vi "cm_Time Domain Display.vi"() -> ()   [LabVIEW 2009, in "Channel Monitor [System].xctl"]
uses:
  Channel Monitor [System].xctl
  <vilib>/Utility/error.llb/DialogType.ctl
panel:
  out "Waveform Graph":waveform(dbl)(graph)
  out "error out":errorcluster
  out "channel":i32
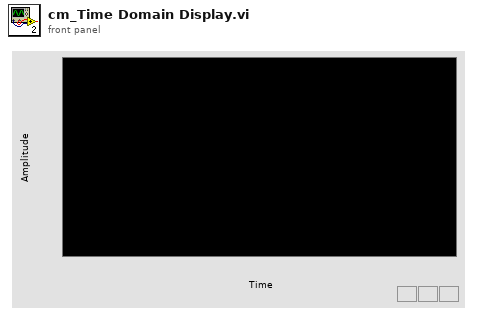
[diagram p1: front panel]
types:
  T1 = typedef "amc_Message Queue.ctl" = refnum<queue>
  T2 = typedef "DialogType.ctl" = u16
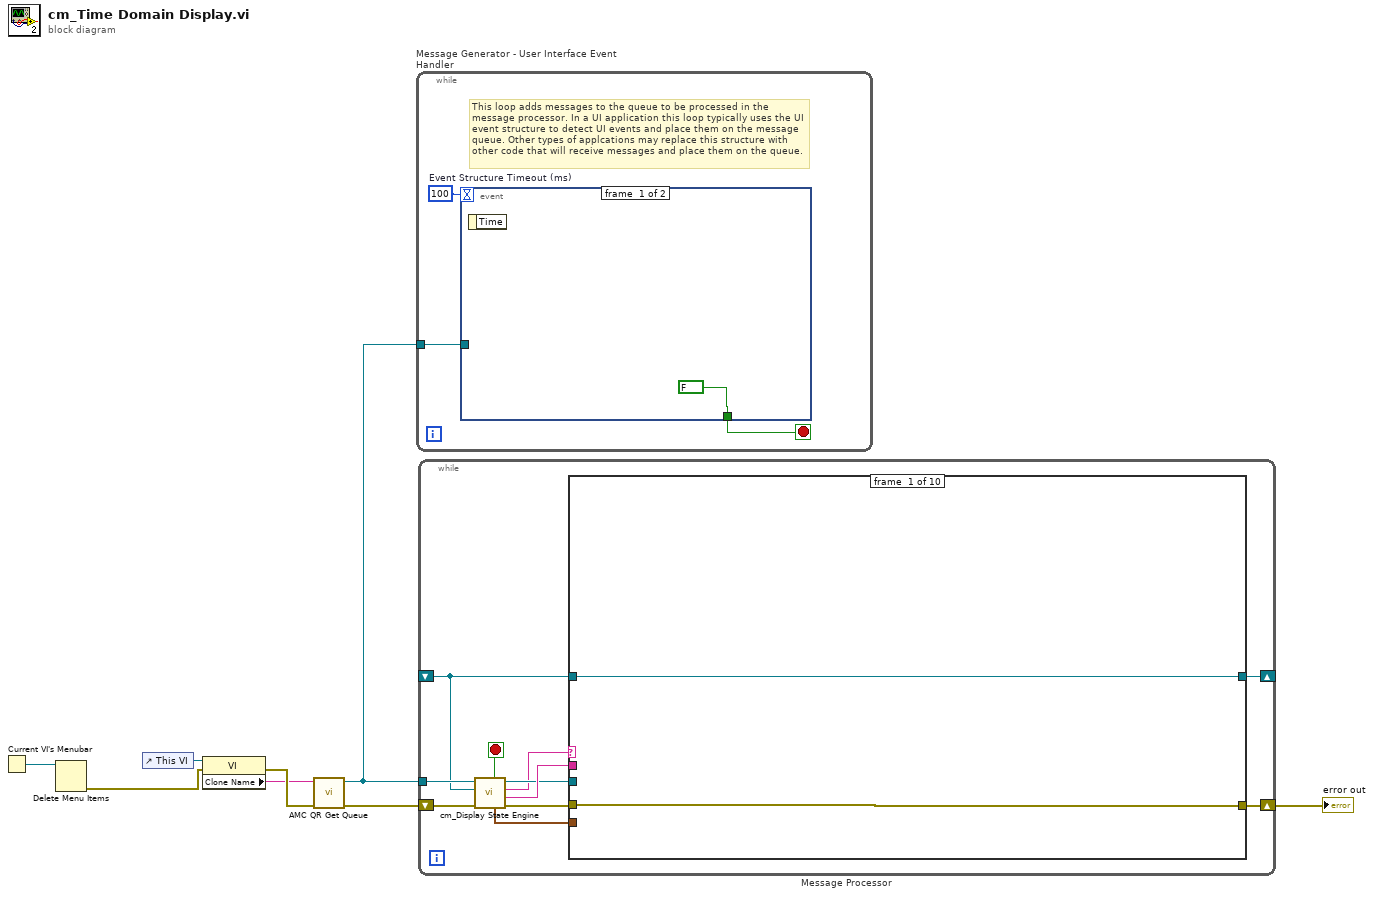
[diagram p0: block diagram]
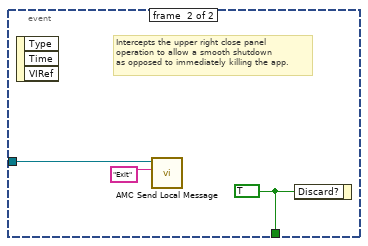
[diagram p2: hidden frame]
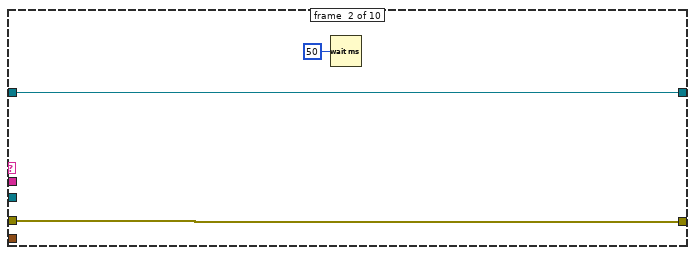
[diagram p3: hidden frame]
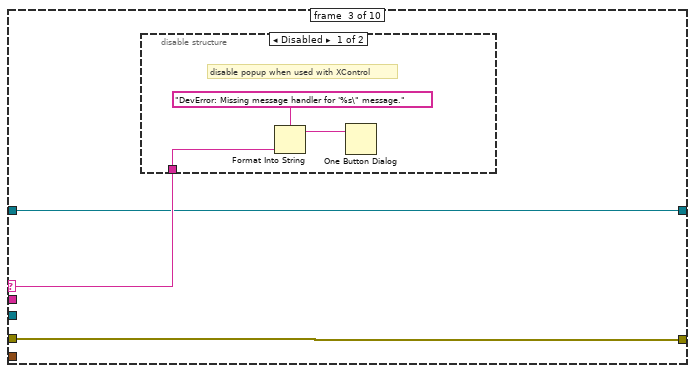
[diagram p4: hidden frame]
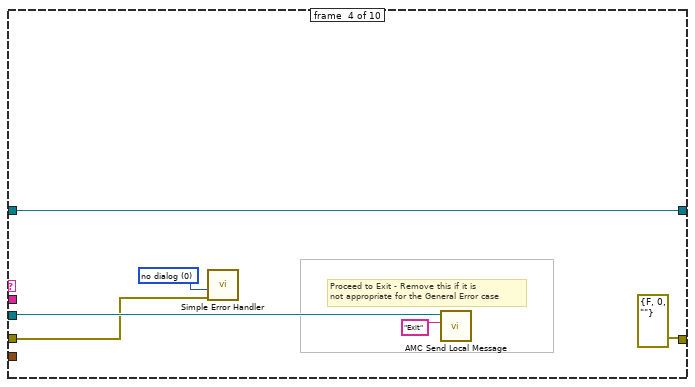
[diagram p6: hidden frame]
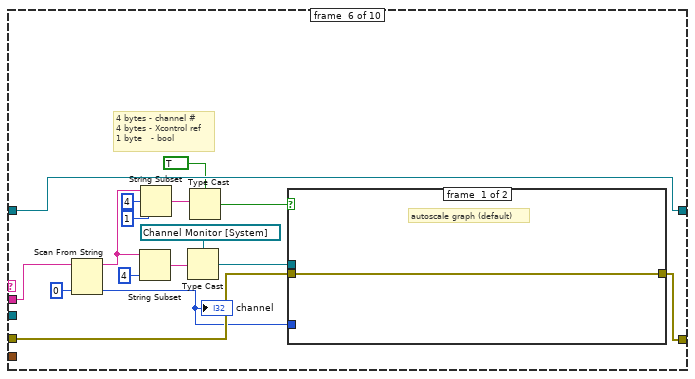
[diagram p8: hidden frame]
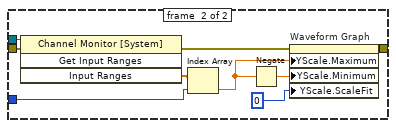
[diagram p9: hidden frame]
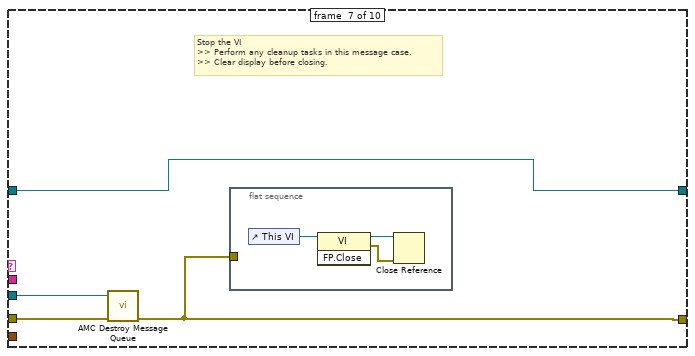
[diagram p10: hidden frame]
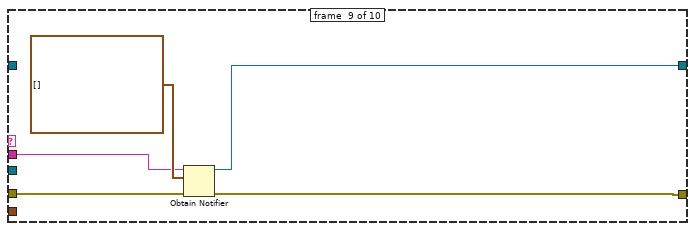
[diagram p12: hidden frame]
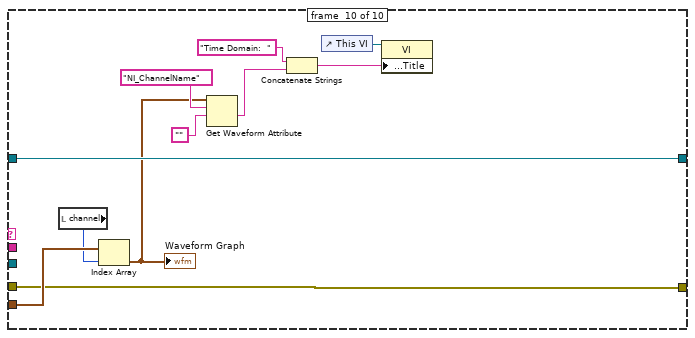
[diagram p13: hidden frame]
diagram:
  n1 = Current VI's Menubar() -> (w6:refnum<k9>)
  n2 = Delete Menu Items(9:w6) -> (0:w4:errorcluster)  [unwired: 3 in, 1 out]
  n3 = control-ref of="This VI"() -> (w7:refnum<vi>)
  n4 = property class="VI"(reference=w7, error in=w4) -> (error out=w5:errorcluster, "Clone Name"=w1:string)  [unwired: 1 out]
  n5 = call <userlib>:"AMC QR Get Queue .vi"("error in (no error)"=w5, "Name"=w1) -> ("error out"=w2:errorcluster, "Queue Out"=w8:T1)  [unwired: 8 in]
  n6 = while "Message Generator - User Interface Event Handler" {
    tunnel: w8 -> [w9]
    stop <- w10 stop-if-true
    w11 = 100  # Event Structure Timeout (ms)
    # "This loop adds messages to the queue to be processed in the message processor. In a UI application this loop typically uses the UI event structure to detect UI events and place them on the message queue. Other types of applcations may replace this structure with other code that will receive messages and place them on the queue."
    n7 = event shown="[1] Panel Close?" {
      selector: _ -> [_ _]
      dyn-events: _ -> [_ _]
      timeout: w11 -> [_ _]
      tunnel: [FALSE w15] -> w10
      tunnel: w9 -> [_ w14]
      event #0 {
        n8 = event-data() -> ()  [unwired: 2 out]
      }
      event #1 {
        w15 = TRUE ("Discard?")
        # "Intercepts the upper right close panel\noperation to allow a smooth shutdown\nas opposed to immediately killing the app."
        n9 = event-data() -> ()  [unwired: 4 out]
        n10 = call <userlib>:"AMC Send Local Message.vi"("Message Name"="Exit", "Message Queue in"=w14) -> ()  [unwired: 4 in, 6 out]
        n11 = event-data("Discard?"=w15) -> ()  [unwired: 1 in, 1 out]
      }
    }
  }
  n12 = while "Message Processor" {
    shift-left: w2 -> [w23]
    shift-right: [w26] -> w3
    tunnel: w8 -> [w24]
    shift-right: [w19] -> _
    shift-left: _ -> [w18]
    stop <- w21 stop-if-true
    n13 = call "cm_Display State Engine.vi"("error in (no error)"=w23, "Wfm Notifier"=w18, "Message Queue"=w24) -> ("error out"=w22:errorcluster, "Message Value"=w25:string, "Message Name"=w16:string, "Message Queue out"=w17:T1, "Data"=w20:waveform(dbl)[], "Exit Process"=w21:bool)  [unwired: 3 in]
    n14 = case shown="\"Initialize\"" w16 {
      selector: w16 -> [_ _ w33 _ _ _ _ _ _ _]
      tunnel: w25 -> [_ _ _ _ _ w55 _ _ w81 _]
      tunnel: w22 -> [w28 w30 w34 w39 w45 w58 w73 w80 w83 w95]
      tunnel: [w28 w30 w34 errorcluster {"status"=FALSE, "code"=0, "source"=""} ("error out") w45 w56 w72 w80 w82 w95] -> w26
      tunnel: w17 -> [_ _ _ w42 _ _ w75 _ _ _]
      tunnel: w20 -> [_ _ _ _ _ _ _ _ _ w96]
      tunnel: [w27 w31 w32 w41 w44 w60 w74 w79 w84 w93] -> w19
      tunnel: w18 -> [w27 w31 w32 w41 w44 w60 w74 w79 _ w93]
      frame #0 {
        # "Dummy case to add a seperator in the Case Structure menu"
      }
      frame #1 {
        n15 = Wait (ms)(milliseconds to wait=u32 50) -> ()  [unwired: 1 out]
      }
      frame #2 {
        # "Call this case if a message is received that is not handled \nby any other case. Typically this is a programming error\nas a result of a typo or unhandled message/missing message handler."
        n16 = disable-structure shown="Disabled" {
          disable-tunnel: w33 -> [w37 _]
          frame #0 {
            # "disable popup when used with XControl"
            n17 = Format Into String(format string="DevError: Missing message handler for '%s\" message." ("message"), w37) -> (resulting string=w35:string)  [unwired: 2 in, 1 out]
            n18 = One Button Dialog(message=w35) -> ()  [unwired: 2 out]
          }
          frame #1 {
          }
        }
      }
      frame #3 {
        w40 = T2 0 items=["no dialog", "OK message", "continue or stop message", "OK message + warnings", "continue/stop + warnings"] ("type of dialog (OK msg:1)")
        # "Proceed to Exit - Remove this if it is\nnot appropriate for the General Error case"
        # "General Error Case - this case is called if an error is passed using the error cluster below. Typically most new errors should be handed in each individual case and not passed in the rror cluster. If necessary a custom error handler case should be added and called from other cases."
        n19 = call <vilib>:"Simple Error Handler.vi"("type of dialog (OK msg:1)"=w40, "error in (no error)"=w39) -> ()  [unwired: 8 out]
        n20 = call <userlib>:"AMC Send Local Message.vi"("Message Name"="Exit", "Message Queue in"=w42) -> ()  [unwired: 4 in, 6 out]
      }
      frame #4 {
        # "Dummy case to add a seperator in the Case Structure menu"
      }
      frame #5 {
        # "4 bytes - channel #\n4 bytes - Xcontrol ref\n1 byte   - bool"
        # "Initialize the state variables and user interface"
        n21 = Scan From String(input string=w55, default 1=0 ("default value 1")) -> (remaining string=w53:string, output 1=w57:i32)  [unwired: 3 in, 2 out]
        "channel" <- w57
        n22 = String Subset(string=w53, length (rest)=4 ("length (rest)")) -> (substring=w54:string)  [unwired: 1 in]
        n23 = String Subset(string=w53, offset (0)=4, length (rest)=1 ("length (rest)")) -> (substring=w48:string)
        n24 = Type Cast(type=refnum<vi> refnum ("Channel Monitor"), x=w54) -> (*(type *) &x=w49:refnum<vi>)
        n25 = Type Cast(type=TRUE, x=w48) -> (*(type *) &x=w46:bool)
        n26 = case shown="True" w46 {
          tunnel: w58 -> [w62 w70]
          tunnel: w57 -> [_ w69]
          tunnel: [w62 w67] -> w56
          tunnel: w49 -> [_ w63]
          frame #0 {
            # "autoscale graph (default)"
          }
          frame #1 {
            n27 = invoke class="Channel Monitor [System]" method="Get Input Ranges"(reference=w63, error in=w70) -> (error out=w68:errorcluster, "Input Ranges"=w71:dbl[])  [unwired: 2 in, 2 out]
            n28 = Index Array(array=w71, index=w69) -> (element=w65:dbl)
            n29 = Negate(x=w65) -> (-x=w66:dbl)
            n30 = property on="Waveform Graph" class="WFGraph (strict)"(error in=w68, "YScale.Maximum"=w65, "YScale.Minimum"=w66, "YScale.ScaleFit"=u8 0 ("Y Scale.Scale Fit")) -> (error out=w67:errorcluster)  [unwired: 1 in, 1 out]
          }
        }
      }
      frame #6 {
        # "Stop the VI\n>> Perform any cleanup tasks in this message case.\n>> Clear display before closing."
        n31 = call <userlib>:"AMC Destroy Message Queue.vi"("error in (no error)"=w73, "Message Queue in"=w75) -> ("error out"=w72:errorcluster)  [unwired: 9 out]
        n32 = flat-sequence {
          tunnel: w72 -> [_]
          frame #0 {
            n33 = control-ref of="This VI"() -> (w76:refnum<vi>)
            n34 = invoke class="VI" method="FP.Close"(reference=w76) -> (reference out=w78:refnum<vi>, error out=w77:errorcluster)  [unwired: 2 in, 1 out]
            n35 = Close Reference(reference=w78, error in (no error)=w77) -> ()  [unwired: 1 out]
          }
        }
      }
      frame #7 {
        # "Dummy case to add a seperator in the Case Structure menu"
      }
      frame #8 {
        n36 = Obtain Notifier(name (unnamed)=w81, notification data type=waveform(dbl)[] [] ("Waveform Graph 2"), error in (no error)=w83) -> (notifier out=w84:refnum<notifier>, error out=w82:errorcluster)  [unwired: 1 in, 1 out]
      }
      frame #9 {
        n37 = local read "channel"() -> (w94:i32)
        n38 = Index Array(array=w96, index=w94) -> (element=w86:waveform(dbl))
        "Waveform Graph" <- w86
        n39 = Get Waveform Attribute(5:"", 6:"NI_ChannelName" ("name"), 7:w86) -> (1:w88:string)  [unwired: 1 in, 3 out]
        n40 = Concatenate Strings("Time Domain:  ", w88) -> (w90:string)
        n41 = control-ref of="This VI"() -> (w92:refnum<vi>)
        n42 = property class="VI"(reference=w92, "Front Panel.Title"=w90) -> ()  [unwired: 1 in, 2 out]
      }
    }
  }
  "error out" <- w3
